vi "close.vi"(8 "error in (no error)":errorcluster, 11 "Stepper in":refnum<class "Stepper.lvclass">) -> (0 "error out":errorcluster, 3 "Stepper out":refnum<class "Stepper.lvclass">)   [LabVIEW 2025, in "Motor.lvlib" / "Stepper.lvclass"]
uses:
  Stepper.lvclass
  Stepper.lvclass/Stepper.ctl
  <vilib>/NI/Modbus Library/API/Master/Modbus Master.lvclass
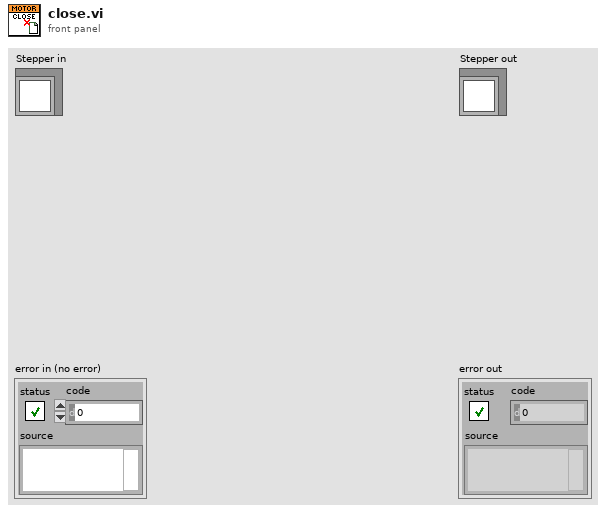
[diagram p1: front panel]
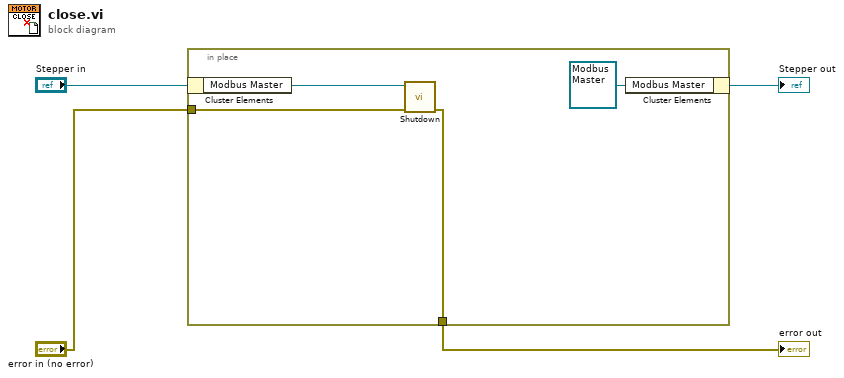
[diagram p0: block diagram]
diagram:
  n1 = in-place {
    in-place-border: [w7] -> w4
    in-place-border: "error in (no error)" -> [w5]
    n2 = in-place-cluster #1("Stepper in") -> ("Modbus Master"=w8:refnum<class "Modbus Master.lvclass">)
    n3 = call-dynamic "Shutdown.vi"("error in"=w5, "Modbus master in"=w8) -> ("error out"=w7:errorcluster)  [unwired: 9 in]
    n4 = in-place-cluster #1("Modbus Master"=refnum<class "Modbus Master.lvclass"> refnum) -> (→"Stepper out":refnum<class "Stepper.lvclass">)
  }
  "error out" <- w4
